vi "Method_Const.vi"(4 "Value":i32, 5 "Input A":refnum<class "Abs_I32 Integer.lvclass">) -> (1 "Result":T1)   [LabVIEW 2021, in "Add_I32.lvclass"]
uses:
  Add_I32.lvclass
  Abs_Types/I32 Integer/Abs_I32 Integer.lvclass
  C:/Program Files (x86)/National Instruments/LabVIEW 2021/vi.lib/TSA/Abstract Data Classes/Abs_Types/Numeric/Abs_Numeric.lvclass
  Abs_Type.ctl
  C:/TSA/LV_Abstract/Source/Functions/Support/Function/Two Terminal/I32/AbsFunc_Two Term_I32.lvclass
  C:/Program Files (x86)/National Instruments/LabVIEW 2021/vi.lib/TSA/Abstract Data Classes/Abs_Types/I32 Integer/Abs_I32 Integer.lvclass
  Support/Function/Two Terminal/I32/AbsFunc_Two Term_I32.lvclass/AbsFunc_Two Term_I32.ctl
  Support/Function/Two Terminal/I32/Properties/Write Numeric A.vi
  Support/Function/Two Terminal/I32/Properties/Write Numeric B.vi
  Constants/Support/I32/Const_I32.lvclass
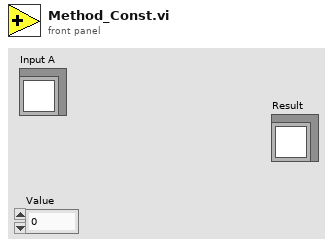
[diagram p1: front panel]
types:
  T1 = typedef "Add_I32.lvclass/Abs_Type.ctl" = refnum<class "Abs_I32 Integer.lvclass">
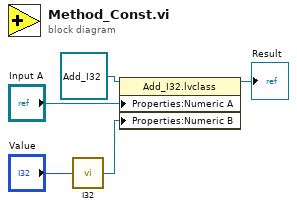
[diagram p0: block diagram]
diagram:
  n1 = call "I32.vi"("Value"="Value") -> ("Constant"=w2:refnum<class "Abs_I32 Integer.lvclass">)  [unwired: 4 in]
  n2 = property class="Add_I32.lvclass"(reference=refnum<class "Add_I32.lvclass"> refnum ("Functions.lvlib:Numeric.lvlib:Add_SGL.lvclass"), "Properties:Numeric A"="Input A", "Properties:Numeric B"=w2) -> (reference out=→"Result":refnum<class "Add_I32.lvclass">)  [unwired: 1 in, 1 out]
